vi "Get Password.vi"(7 "IonSniffer777":string="IonSniffer777") -> (1 "Advanced":bool, 3 "Valid":bool)   [LabVIEW 2015]
panel:
  in  "Remember My Password":bool
  in  "Password":string
  in  "Done":bool
  # "Please enter a valid password in order to access the selected feature.\n(note the password is case sensitive)"
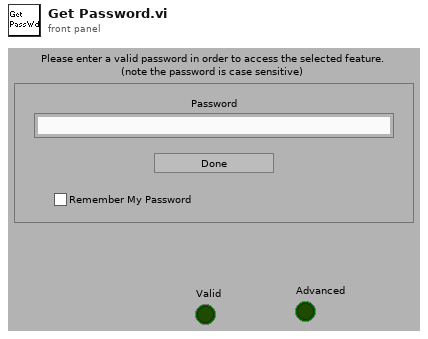
[diagram p1: front panel]
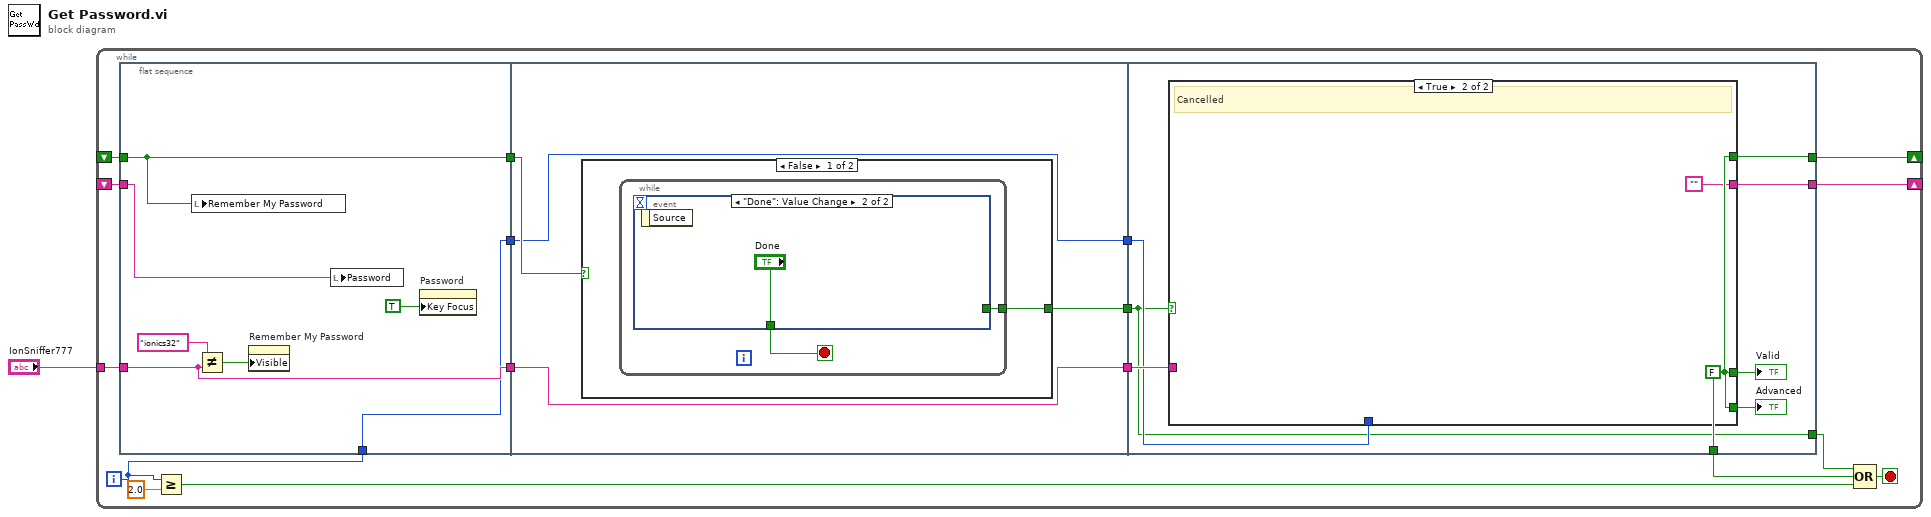
[diagram p0: block diagram]
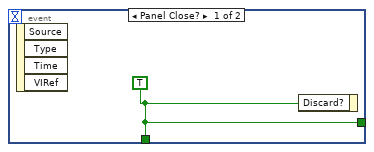
[diagram p2: hidden frame]
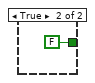
[diagram p3: hidden frame]
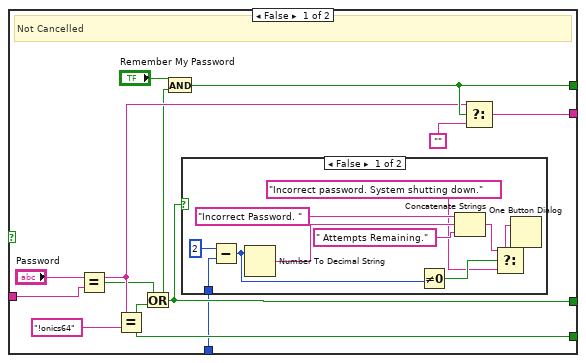
[diagram p4: hidden frame]
diagram:
  n1 = while {
    shift-right: [w18] -> _
    shift-left: _ -> [w17]
    shift-right: [w16] -> _
    shift-left: _ -> [w15]
    tunnel: "IonSniffer777" -> [w14]
    i -> [w9]
    stop <- w12 stop-if-true
    n2 = flat-sequence {
      tunnel: w17 -> [w24]
      tunnel: [w24] -> w7
      tunnel: w15 -> [w23]
      tunnel: w14 -> [w22]
      tunnel: [w22] -> w6
      tunnel: w9 -> [w19]
      tunnel: [w19] -> w5
      tunnel: w7 -> [w29]
      tunnel: w6 -> [w27]
      tunnel: [w27] -> w4
      tunnel: w5 -> [w26]
      tunnel: [w26] -> w3
      tunnel: [w28] -> w2
      tunnel: [w42] -> w18
      tunnel: [w41] -> w16
      tunnel: w4 -> [w40]
      tunnel: [w38] -> w13
      tunnel: w3 -> [w37]
      tunnel: [w36] -> w8
      tunnel: w2 -> [w36]
      frame #0 {
        n3 = local write "Remember My Password"(w24) -> ()
        n4 = Not Equal?(x="ionics32" ("IonSniffer777"), y=w22) -> (x != y?=w20:bool)
        n5 = property on="Remember My Password" class="Bool (strict)"("Visible"=w20) -> ()  [unwired: 2 in, 2 out]
        n6 = local write "Password"(w23) -> ()
        n7 = property on="Password" class="Str"("Key Focus"=TRUE) -> ()  [unwired: 2 in, 2 out]
      }
      frame #1 {
        n8 = case shown="False" w29 {
          tunnel: [w30 FALSE] -> w28
          frame False {
            n9 = while {
              tunnel: [w31] -> w30
              stop <- w32 stop-if-true
              n10 = event shown="[1] \"Done\": Value Change" {
                selector: _ -> [_ _]
                dyn-events: _ -> [_ _]
                timeout: _ -> [_ _]
                tunnel: [w33 "Done"] -> w32
                tunnel: [w33 _] -> w31
                event Panel Close? {
                  w33 = TRUE
                  n11 = event-data() -> ()  [unwired: 5 out]
                  n12 = event-data("Discard?"=w33) -> ()  [unwired: 1 in, 1 out]
                }
                event "Done": Value Change {
                  n13 = event-data() -> ()  [unwired: 2 out]
                }
              }
            }
          }
          frame True {
          }
        }
      }
      frame #2 {
        n14 = case shown="True" w36 {
          tunnel: [w52 w65] -> w42
          tunnel: [w50 ""] -> w41
          tunnel: w40 -> [w49 _]
          tunnel: [w45 w65] -> w39
          tunnel: [w44 w65] -> w38
          tunnel: w37 -> [w43 _]
          frame False {
            # "Not Cancelled"
            n15 = Equal?(x="Password", y=w49) -> (x = y?=w46:bool)
            n16 = Equal?(x="Password", y="!onics64") -> (x = y?=w45:bool)
            n17 = Or(x=w46, y=w45) -> (x .or. y?=w44:bool)
            n18 = And(x="Remember My Password", y=w44) -> (x .and. y?=w52:bool)
            n19 = case shown="False" w44 {
              tunnel: w43 -> [w59 _]
              frame False {
                n20 = Subtract(x=2 ("y"), y=w59) -> (x-y=w55:i32)
                n21 = Number To Decimal String(number=w55) -> (decimal integer string=w61:string)  [unwired: 1 in]
                n22 = Not Equal To 0?(x=w55) -> (x != 0?=w58:bool)
                n23 = Concatenate Strings("Incorrect Password. " ("message"), w61, " Attempts Remaining." ("string")) -> (w57:string)
                n24 = Select(t=w57, s=w58, f="Incorrect password. System shutting down.") -> (s? t:f=w54:string)
                n25 = One Button Dialog(message=w54) -> ()  [unwired: 1 in, 1 out]
              }
              frame True {
              }
            }
            n26 = Select(t="Password", s=w52, f="") -> (s? t:f=w50:string)
          }
          frame True {
            w65 = FALSE
            # "Cancelled"
          }
        }
        "Valid" <- w38
        "Advanced" <- w39
      }
    }
    n27 = Greater Or Equal?(x=w9, y=2.0) -> (x >= y?=w10:bool)
    n28 = Compound Arithmetic op=OR(w8, w13, w10) -> (w12:bool)
  }
